vi "Set Value on Multiple Controls.vi"(10 "Enable?":bool, 11 "Controls":refnum<vi>[](array[refnum])) -> ()   [LabVIEW 2019, in "CML UI.lvlib"]
doc: "Sets all the controls in the input array to the \"Enable state\" value.\n_____\nBased on DQMH Project Template 6.1.0.94."
uses:
  CML UI.lvlib
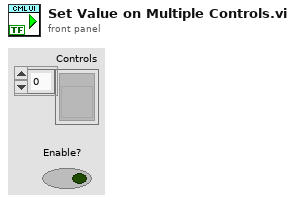
[diagram p1: front panel]
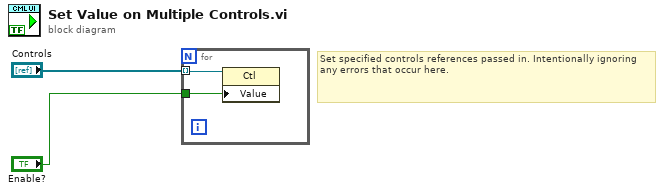
[diagram p0: block diagram]
diagram:
  # "Set specified controls references passed in. Intentionally ignoring any errors that occur here."
  n1 = for {
    tunnel: "Controls" -> [w4] mode=indexing
    tunnel: "Enable?" -> [w3]
    n2 = property on="Property Node" class="Ctl"(reference=w4, "Value"=w3) -> ()  [unwired: 1 in, 2 out]
  }
